vi "Field Draw Ball.vi"(3 "Project":T1=enum."VSS", 4 "Draw Targets?":T2, 6 "Lado":enum16{"Esquerdo", "Direito"}(ring), 7 "Referee":refnum<class "Referee.lvclass">, 8 "picture in":picture, 9 "Offset":T3, 10 "Scale mm/pixel":dbl, 11 "BallRef":refnum<class "Ball.lvclass">) -> (0 "picture out":picture)   [LabVIEW 2020]
uses:
  <vilib>/Utility/miscctls.llb/LVBoundsTypeDef.ctl
  DrawTargets.ctl
  Ball_class/Ball.lvclass
  Parameters_class/Project.ctl
  Referee_class/Referee.lvclass
  Object_class/Object.lvclass/Object.ctl
  Object_class/Read x.vi
  Object_class/Read y.vi
  Object_class/Read pos_est_x.vi
  Object_class/Read pos_est_y.vi
  <vilib>/Analysis/NI_AALPro.lvlib
  <vilib>/Analysis/coordinate.llb/2D Cartesian Coordinate Rotation (Scalar).vi
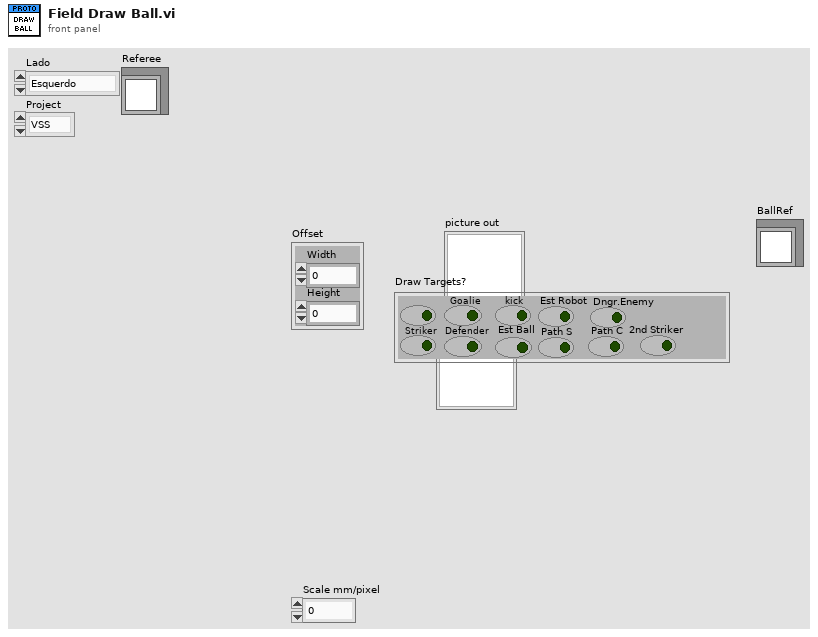
[diagram p1: front panel]
types:
  T1 = typedef "Project.ctl" = enum16{"SSL", "VSS"}
  T2 = typedef "DrawTargets.ctl" = cluster{"Attacker":bool, "Striker":bool, "Goalie":bool, "Defender":bool, "kick":bool, "Est Ball":bool, "Est Robot":bool, "Path S":bool, "Path C":bool, "Dngr.Enemy":bool, "2nd Striker":bool}
  T3 = typedef "LVBoundsTypeDef.ctl" = cluster{"Width":u32, "Height":u32}
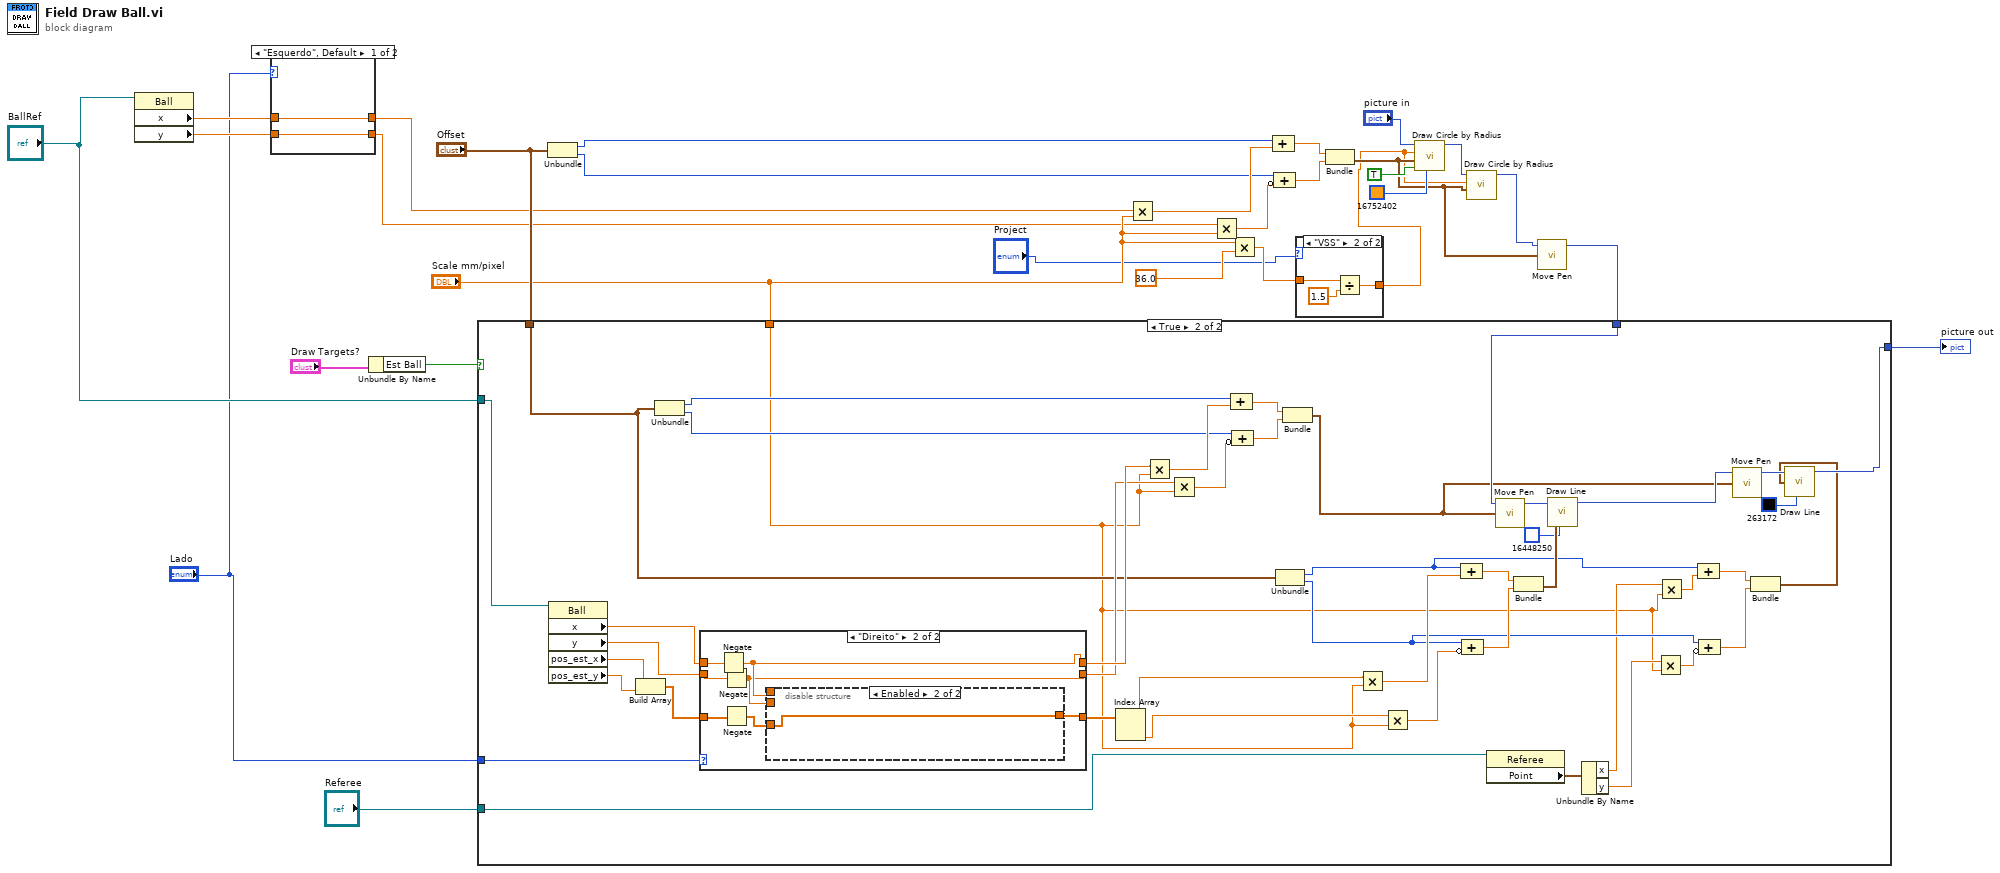
[diagram p0: block diagram]
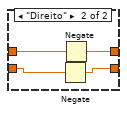
[diagram p3: hidden frame]
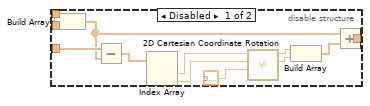
[diagram p6: hidden frame]
diagram:
  n1 = property class="Ball"(reference="BallRef") -> ("x"=w7:dbl, "y"=w6:dbl)  [unwired: 1 in, 2 out]
  n2 = case shown="\"Esquerdo\", Default" "Lado" {
    tunnel: [w31 w35] -> w9
    tunnel: w7 -> [w31 w32]
    tunnel: [w30 w33] -> w8
    tunnel: w6 -> [w30 w34]
    frame "Esquerdo", Default {
    }
    frame "Direito" {
      n3 = Negate(x=w34) -> (-x=w33:dbl)
      n4 = Negate(x=w32) -> (-x=w35:dbl)
    }
  }
  n5 = Unbundle By Name("Draw Targets?") -> ("Est Ball"=w11:bool)
  n6 = Unbundle("Offset") -> ("Width"=w26:u32, "Height"=w23:u32)
  n7 = Multiply(x=w9, y="Scale mm/pixel") -> (x*y=w25:dbl)
  n8 = Multiply(x=w8, y="Scale mm/pixel") -> (x*y=w22:dbl)
  n9 = Multiply(x="Scale mm/pixel", y=sgl 36.0 ("radius")) -> (x*y=w4:dbl)
  n10 = Compound Arithmetic op=ADD(w26, w25) -> (w24:dbl)
  n11 = Compound Arithmetic op=ADD(w23, invert w22) -> (w21:dbl)
  n12 = case shown="\"VSS\"" "Project" {
    tunnel: w4 -> [w36 w39]
    tunnel: [w36 w37] -> w3
    frame "SSL", Default {
    }
    frame "VSS" {
      n13 = Divide(x=w39, y=1.5) -> (x/y=w37:dbl)
    }
  }
  n14 = Bundle(w24, w21) -> (w15:cluster{dbl, dbl})  [unwired: 1 in]
  n15 = call <vilib>:"Draw Circle by Radius.vi"("color(black)"=u32 16752402, "fill?(F)"=TRUE, "pixel center"=w15, "radius"=w3, "picture"="picture in") -> ("new picture"=w19:picture)  [unwired: 6 in]
  n16 = call <vilib>:"Draw Circle by Radius.vi"("pixel center"=w15, "radius"=w3, "picture"=w19) -> ("new picture"=w16:picture)  [unwired: 8 in]
  n17 = call <vilib>:"Move Pen.vi"("new position"=w15, "picture"=w16) -> ("new picture"=w17:picture)  [unwired: 3 in]
  n18 = case shown="True" w11 {
    tunnel: [w40 w48] -> w18
    tunnel: w17 -> [w40 w59]
    tunnel: "Offset" -> [_ w61]
    tunnel: "Scale mm/pixel" -> [_ w43]
    tunnel: "BallRef" -> [_ w60]
    tunnel: "Lado" -> [_ w58]
    tunnel: "Referee" -> [_ w53]
    frame False {
    }
    frame True {
      n19 = property class="Ball"(reference=w60) -> ("x"=w62:dbl, "y"=w63:dbl, "pos_est_x"=w66:dbl, "pos_est_y"=w65:dbl)  [unwired: 1 in, 2 out]
      n20 = Build Array(w66, w65) -> (w64:dbl[])
      n21 = Unbundle(w61) -> ("Width"=w84:u32, "Height"=w81:u32)
      n22 = case shown="\"Direito\"" w58 {
        tunnel: [w87 w91] -> w69
        tunnel: w62 -> [w87 w94]
        tunnel: [w86 w90] -> w68
        tunnel: w63 -> [w86 w93]
        tunnel: [w85 w88] -> w67
        tunnel: w64 -> [w85 w92]
        frame "Esquerdo", Default {
        }
        frame "Direito" {
          n23 = Negate(x=w94) -> (-x=w91:dbl)
          n24 = Negate(x=w93) -> (-x=w90:dbl)
          n25 = Negate(x=w92) -> (-x=w89:dbl[])
          n26 = disable-structure shown="Enabled" {
            disable-tunnel: w91 -> [w101 _]
            disable-tunnel: w90 -> [w100 _]
            disable-tunnel: w89 -> [w99 w107]
            disable-tunnel: [w97 w107] -> w88
            frame Disabled {
              n27 = Build Array(w101, w100) -> (w95:dbl[])
              n28 = Subtract(x=w99, y=w95) -> (x-y=w98:dbl[])
              n29 = Index Array(array=w98) -> (element #1=w106:dbl, element #2=w105:dbl)  [unwired: 2 in]
              n30 = call-poly <vilib>:"2D Cartesian Coordinate Rotation.vi"("theta"=3.141592653589793, "y"=w105, "x"=w106) -> ("y out"=w103:dbl, "x out"=w104:dbl)  [unwired: 6 in, 1 out]
              n31 = Build Array(w104, w103) -> (w96:dbl[])
              n32 = Add(x=w95, y=w96) -> (x+y=w97:dbl[])
            }
            frame Enabled {
            }
          }
        }
      }
      n33 = Index Array(array=w67) -> (element #1=w72:dbl, element #2=w71:dbl)  [unwired: 2 in]
      n34 = Multiply(x=w69, y=w43) -> (x*y=w83:dbl)
      n35 = Multiply(x=w68, y=w43) -> (x*y=w80:dbl)
      n36 = Compound Arithmetic op=ADD(w84, w83) -> (w82:dbl)
      n37 = Compound Arithmetic op=ADD(w81, invert w80) -> (w79:dbl)
      n38 = Unbundle(w61) -> ("Width"=w55:u32, "Height"=w54:u32)
      n39 = Bundle(w82, w79) -> (w47:cluster{dbl, dbl})  [unwired: 1 in]
      n40 = Multiply(x=w72, y=w43) -> (x*y=w74:dbl)
      n41 = Multiply(x=w71, y=w43) -> (x*y=w73:dbl)
      n42 = Compound Arithmetic op=ADD(w55, w74) -> (w77:dbl)
      n43 = Compound Arithmetic op=ADD(w54, invert w73) -> (w76:dbl)
      n44 = property class="Referee"(reference=w53) -> ("Point"=w52:cluster{"x":sgl, "y":sgl})  [unwired: 1 in, 2 out]
      n45 = call <vilib>:"Move Pen.vi"("new position"=w47, "picture"=w59) -> ("new picture"=w78:picture)  [unwired: 3 in]
      n46 = Bundle(w77, w76) -> (w75:cluster{dbl, dbl})  [unwired: 1 in]
      n47 = call <vilib>:"Draw Line.vi"("picture"=w78, "end point"=w75, "color(black)"=u32 16448250) -> ("new picture"=w49:picture)  [unwired: 6 in]
      n48 = Unbundle By Name(w52) -> ("x"=w45:sgl, "y"=w44:sgl)
      n49 = Multiply(x=w44, y=w43) -> (x*y=w41:dbl)
      n50 = Multiply(x=w45, y=w43) -> (x*y=w42:dbl)
      n51 = Compound Arithmetic op=ADD(w55, w42) -> (w57:dbl)
      n52 = Compound Arithmetic op=ADD(w54, invert w41) -> (w56:dbl)
      n53 = call <vilib>:"Move Pen.vi"("new position"=w47, "picture"=w49) -> ("new picture"=w50:picture)  [unwired: 3 in]
      n54 = Bundle(w57, w56) -> (w46:cluster{dbl, dbl})  [unwired: 1 in]
      n55 = call <vilib>:"Draw Line.vi"("picture"=w50, "end point"=w46, "color(black)"=u32 263172) -> ("new picture"=w48:picture)  [unwired: 6 in]
    }
  }
  "picture out" <- w18
